vi "Server.vi"() -> ()   [LabVIEW 2021]
panel:
  out "MasterBedRoomD":u8(slide) scale=0.0..100.0
  out "Balcony2D":u8(slide) scale=0.0..100.0
  out "KitchenToiletD":u8(slide) scale=0.0..100.0
  out "Balcony1D2":u8(slide) scale=0.0..100.0
  out "LivingRoomD":u8(slide) scale=0.0..100.0
  out "LRToiletD":u8(slide) scale=0.0..100.0
  out "KitchenD":u8(slide) scale=0.0..100.0
  out "Balcony1D1":u8(slide) scale=0.0..100.0
  out "MBToiletD":u8(slide) scale=0.0..100.0
  out "Bedroom1D":u8(slide) scale=0.0..100.0
  out "Bedroom2D":u8(slide) scale=0.0..100.0
  out "MasterBedroomL2":bool
  out "MasterBedroomL1":bool
  out "LivingRoomL2":bool
  out "Bedroom1L":bool
  out "Bedroom2L":bool
  out "LRToiletL":bool
  out "LivingRoomL1":bool
  out "KitchenToiletL":bool
  out "KitchenL":bool
  out "BalconyL3":bool
  out "BalconyL2":bool
  out "BalconyL1":bool
  out "LivingRoomC":u8(slide) scale=0.0..10.0
  out "MasterBedroomC":u8(slide) scale=0.0..10.0
  in  "WindowsMediaPlayer":refnum<k7>(container)
  out "Electric Usage":dbl(knob) scale=0.0..100.0
  # "Balcony 2"
  # "TV"
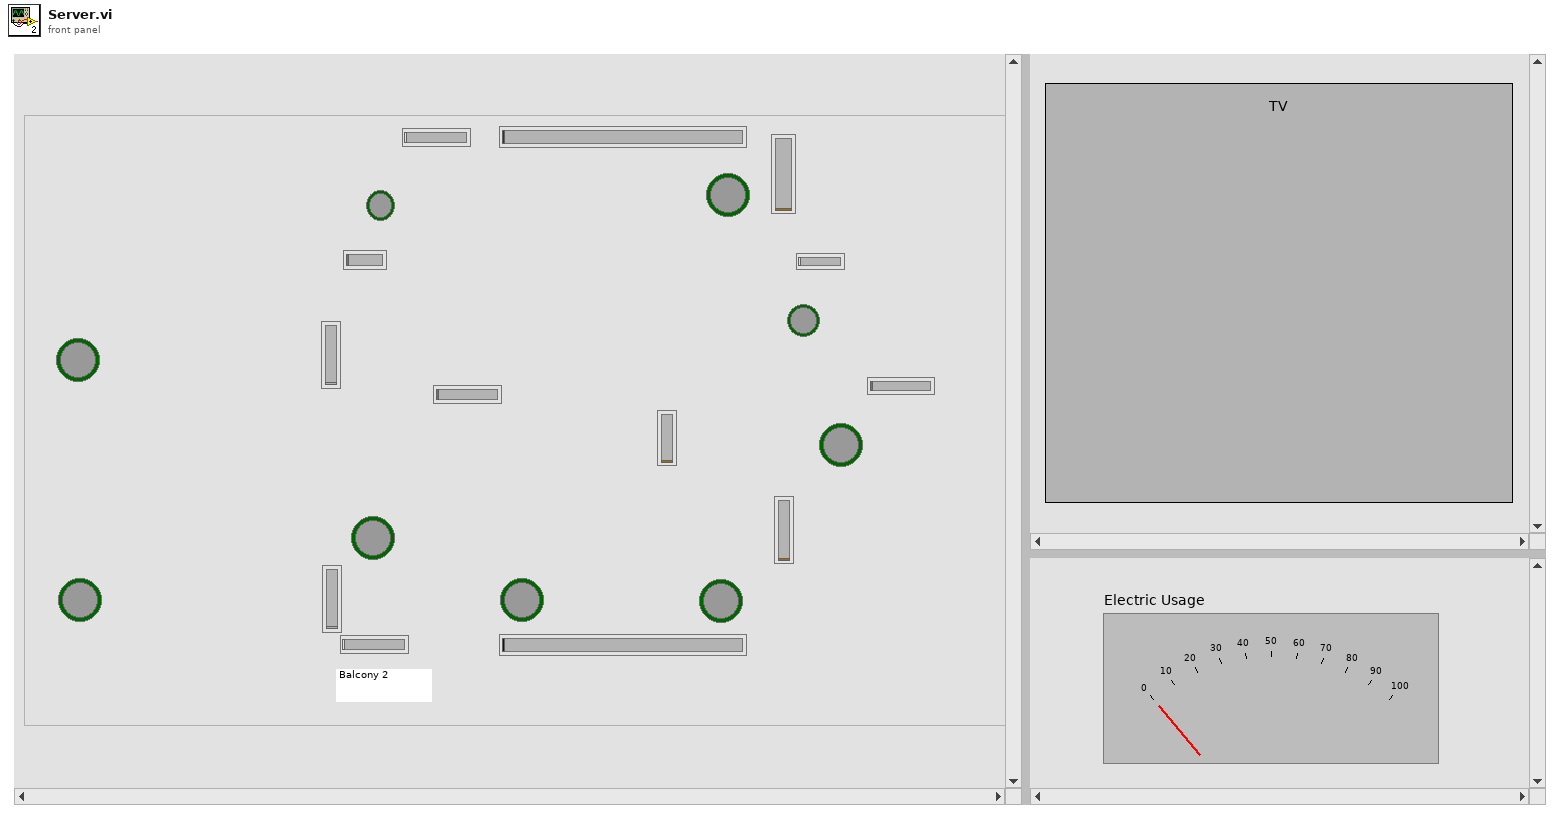
[diagram p1: front panel]
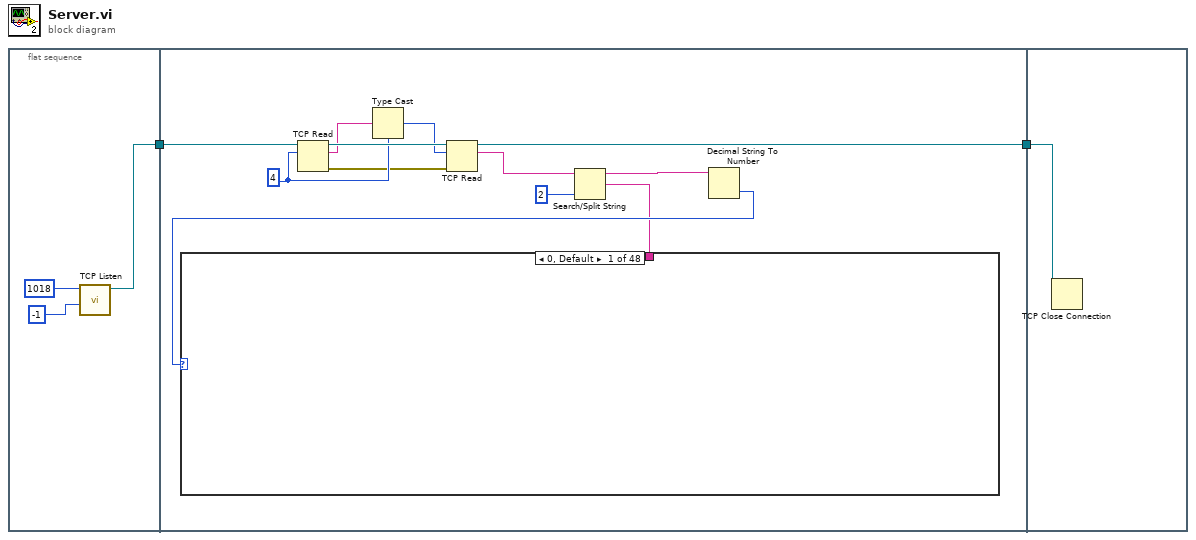
[diagram p0: block diagram]
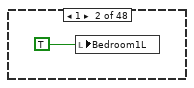
[diagram p2: hidden frame]
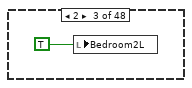
[diagram p3: hidden frame]
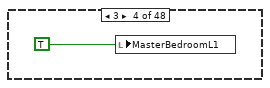
[diagram p4: hidden frame]
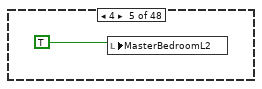
[diagram p5: hidden frame]
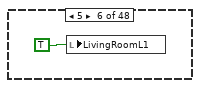
[diagram p6: hidden frame]
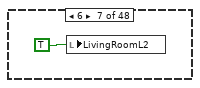
[diagram p7: hidden frame]
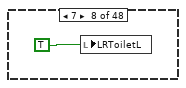
[diagram p8: hidden frame]
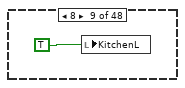
[diagram p9: hidden frame]
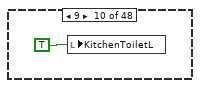
[diagram p10: hidden frame]
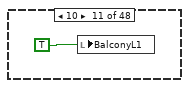
[diagram p11: hidden frame]
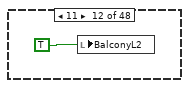
[diagram p12: hidden frame]
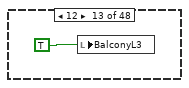
[diagram p13: hidden frame]
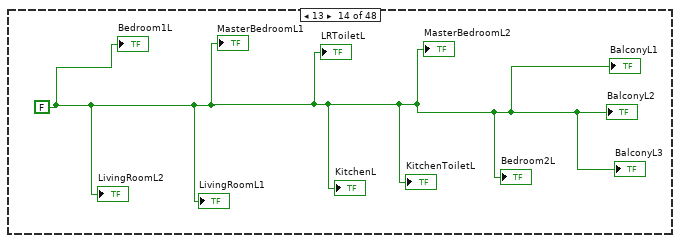
[diagram p14: hidden frame]
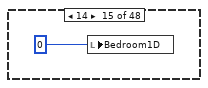
[diagram p15: hidden frame]
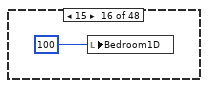
[diagram p16: hidden frame]
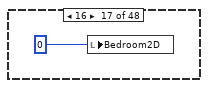
[diagram p17: hidden frame]
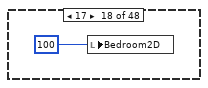
[diagram p18: hidden frame]
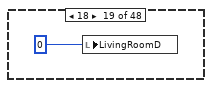
[diagram p19: hidden frame]
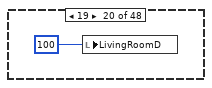
[diagram p20: hidden frame]
diagram:
  n1 = flat-sequence {
    tunnel: [w4] -> w2
    tunnel: w2 -> [w13]
    tunnel: [w12] -> w1
    tunnel: w1 -> [w95]
    frame #0 {
      n2 = call <vilib>:"TCP Listen.vi"("timeout ms (wait forever: -1)"=-1, "port"=1018) -> ("connection ID"=w4:refnum<k5>)  [unwired: 5 in, 4 out]
    }
    frame #1 {
      w11 = 4
      n3 = TCP Read(connection ID=w13, bytes to read=w11) -> (connection ID out=w17:refnum<k5>, data out=w15:string, error out=w6:errorcluster)  [unwired: 3 in]
      n4 = Type Cast(type=w11, x=w15) -> (*(type *) &x=w16:i32)
      n5 = TCP Read(connection ID=w17, bytes to read=w16, error in (no error)=w6) -> (connection ID out=w12:refnum<k5>, data out=w8:string)  [unwired: 2 in, 1 out]
      n6 = Search/Split String(string=w8, offset (0)=2) -> (substring before match=w7:string, match + rest of string=w9:string)  [unwired: 1 in, 1 out]
      n7 = Decimal String To Number(string=w7) -> (number=w10:i32)  [unwired: 2 in, 1 out]
      n8 = case shown="0, Default" w10 {
        tunnel: w9 -> [_ _ _ _ _ _ _ _ _ _ _ _ _ _ _ _ _ _ _ _ _ _ _ _ _ _ _ _ _ _ _ _ _ _ _ _ _ w55 w57 _ _ _ _ _ _ w82 w93 _]
        frame 0, Default {
        }
        frame 1 {
          n9 = local write "Bedroom1L"(TRUE) -> ()
        }
        frame 2 {
          n10 = local write "Bedroom2L"(TRUE) -> ()
        }
        frame 3 {
          n11 = local write "MasterBedroomL1"(TRUE) -> ()
        }
        frame 4 {
          n12 = local write "MasterBedroomL2"(TRUE) -> ()
        }
        frame 5 {
          n13 = local write "LivingRoomL1"(TRUE) -> ()
        }
        frame 6 {
          n14 = local write "LivingRoomL2"(TRUE) -> ()
        }
        frame 7 {
          n15 = local write "LRToiletL"(TRUE) -> ()
        }
        frame 8 {
          n16 = local write "KitchenL"(TRUE) -> ()
        }
        frame 9 {
          n17 = local write "KitchenToiletL"(TRUE) -> ()
        }
        frame 10 {
          n18 = local write "BalconyL1"(TRUE) -> ()
        }
        frame 11 {
          n19 = local write "BalconyL2"(TRUE) -> ()
        }
        frame 12 {
          n20 = local write "BalconyL3"(TRUE) -> ()
        }
        frame 13 {
          w30 = FALSE
          "BalconyL1" <- w30
          "KitchenToiletL" <- w30
          "LivingRoomL1" <- w30
          "LRToiletL" <- w30
          "Bedroom1L" <- w30
          "LivingRoomL2" <- w30
          "MasterBedroomL1" <- w30
          "MasterBedroomL2" <- w30
          "BalconyL3" <- w30
          "KitchenL" <- w30
          "BalconyL2" <- w30
          "Bedroom2L" <- w30
        }
        frame 14 {
          n21 = local write "Bedroom1D"(0) -> ()
        }
        frame 15 {
          n22 = local write "Bedroom1D"(100) -> ()
        }
        frame 16 {
          n23 = local write "Bedroom2D"(0) -> ()
        }
        frame 17 {
          n24 = local write "Bedroom2D"(100) -> ()
        }
        frame 18 {
          n25 = local write "LivingRoomD"(0) -> ()
        }
        frame 19 {
          n26 = local write "LivingRoomD"(100) -> ()
        }
        frame 20 {
          n27 = local write "LRToiletD"(0) -> ()
        }
        frame 21 {
          n28 = local write "LRToiletD"(100) -> ()
        }
        frame 22 {
          n29 = local write "MasterBedRoomD"(0) -> ()
        }
        frame 23 {
          n30 = local write "MasterBedRoomD"(100) -> ()
        }
        frame 24 {
          n31 = local write "MBToiletD"(0) -> ()
        }
        frame 25 {
          n32 = local write "MBToiletD"(100) -> ()
        }
        frame 26 {
          n33 = local write "KitchenD"(0) -> ()
        }
        frame 27 {
          n34 = local write "KitchenD"(100) -> ()
        }
        frame 28 {
          n35 = local write "KitchenToiletD"(0) -> ()
        }
        frame 29 {
          n36 = local write "KitchenToiletD"(100) -> ()
        }
        frame 30 {
          n37 = local write "Balcony1D1"(0) -> ()
        }
        frame 31 {
          n38 = local write "Balcony1D1"(100) -> ()
        }
        frame 32 {
          n39 = local write "Balcony1D2"(0) -> ()
        }
        frame 33 {
          n40 = local write "Balcony1D2"(100) -> ()
        }
        frame 34 {
          n41 = local write "Balcony2D"(0) -> ()
        }
        frame 35 {
          n42 = local write "Balcony2D"(100) -> ()
        }
        frame 36 {
          w53 = 100
          "Balcony2D" <- w53
          "Bedroom1D" <- w53
          "Bedroom2D" <- w53
          "MasterBedRoomD" <- w53
          "MBToiletD" <- w53
          "Balcony1D1" <- w53
          "Balcony1D2" <- w53
          "LRToiletD" <- w53
          "LivingRoomD" <- w53
          "KitchenD" <- w53
          "KitchenToiletD" <- w53
        }
        frame 37 {
          n43 = Decimal String To Number(string=w55) -> (number=→"LivingRoomC":i32)  [unwired: 2 in, 1 out]
        }
        frame 38 {
          n44 = Decimal String To Number(string=w57) -> (number=→"MasterBedroomC":i32)  [unwired: 2 in, 1 out]
        }
        frame 39 {
          n45 = Automation Open(Automation Refnum="WindowsMediaPlayer") -> (Automation Refnum=w60:refnum<k7>)  [unwired: 3 in, 1 out]
          n46 = property class="IWMPPlayer4"(reference=w60) -> ("controls"=w59:refnum<k7>)  [unwired: 1 in, 2 out]
          n47 = invoke class="IWMPControls" method="stop"(reference=w59) -> (reference out=w58:refnum<k7>)  [unwired: 2 in, 2 out]
          n48 = Close Reference(reference=w58) -> ()  [unwired: 1 in, 1 out]
        }
        frame 40 {
          # "Pause"
          n49 = local read "WindowsMediaPlayer"() -> (w62:refnum<k7>)
          n50 = Automation Open(Automation Refnum=w62) -> (Automation Refnum=w63:refnum<k7>)  [unwired: 3 in, 1 out]
          n51 = property class="IWMPPlayer4"(reference=w63) -> ("controls"=w64:refnum<k7>)  [unwired: 1 in, 2 out]
          n52 = invoke class="IWMPControls" method="pause"(reference=w64) -> (reference out=w65:refnum<k7>)  [unwired: 2 in, 2 out]
          n53 = Close Reference(reference=w65) -> ()  [unwired: 1 in, 1 out]
        }
        frame 41 {
          # "Channel1"
          n54 = local read "WindowsMediaPlayer"() -> (w67:refnum<k7>)
          n55 = Automation Open(Automation Refnum=w67) -> (Automation Refnum=w68:refnum<k7>)  [unwired: 3 in, 1 out]
          n56 = property class="IWMPPlayer4"(reference=w68, "URL"="D:\\APU\\Academics\\Degree\\Year 2 - Sem 1\\spcc\\Assignment\\Submission\\YamChenXi_TP061635\\Materials\\Advert.mp4") -> (reference out=w69:refnum<k7>)  [unwired: 1 in, 1 out]
          n57 = Close Reference(reference=w69) -> ()  [unwired: 1 in, 1 out]
        }
        frame 42 {
          # "Channel2"
          n58 = local read "WindowsMediaPlayer"() -> (w73:refnum<k7>)
          n59 = Automation Open(Automation Refnum=w73) -> (Automation Refnum=w72:refnum<k7>)  [unwired: 3 in, 1 out]
          n60 = property class="IWMPPlayer4"(reference=w72, "URL"="D:\\APU\\Academics\\Degree\\Year 2 - Sem 1\\spcc\\Assignment\\Submission\\YamChenXi_TP061635\\Materials\\Wildlife.mp4") -> (reference out=w71:refnum<k7>)  [unwired: 1 in, 1 out]
          n61 = Close Reference(reference=w71) -> ()  [unwired: 1 in, 1 out]
        }
        frame 43 {
          # "Channel3"
          n62 = local read "WindowsMediaPlayer"() -> (w77:refnum<k7>)
          n63 = Automation Open(Automation Refnum=w77) -> (Automation Refnum=w76:refnum<k7>)  [unwired: 3 in, 1 out]
          n64 = property class="IWMPPlayer4"(reference=w76, "URL"="D:\\APU\\Academics\\Degree\\Year 2 - Sem 1\\spcc\\Assignment\\Submission\\YamChenXi_TP061635\\Materials\\CuriousCat.mp4") -> (reference out=w75:refnum<k7>)  [unwired: 1 in, 1 out]
          n65 = Close Reference(reference=w75) -> ()  [unwired: 1 in, 1 out]
        }
        frame 44 {
          # "Play"
          n66 = local read "WindowsMediaPlayer"() -> (w81:refnum<k7>)
          n67 = Automation Open(Automation Refnum=w81) -> (Automation Refnum=w80:refnum<k7>)  [unwired: 3 in, 1 out]
          n68 = property class="IWMPPlayer4"(reference=w80) -> ("controls"=w79:refnum<k7>)  [unwired: 1 in, 2 out]
          n69 = invoke class="IWMPControls" method="play"(reference=w79) -> (reference out=w78:refnum<k7>)  [unwired: 2 in, 2 out]
          n70 = Close Reference(reference=w78) -> ()  [unwired: 1 in, 1 out]
        }
        frame 45 {
          # "Volume"
          n71 = local read "WindowsMediaPlayer"() -> (w87:refnum<k7>)
          n72 = Automation Open(Automation Refnum=w87) -> (Automation Refnum=w83:refnum<k7>)  [unwired: 3 in, 1 out]
          n73 = property class="IWMPPlayer4"(reference=w83) -> ("settings"=w84:refnum<k7>)  [unwired: 1 in, 2 out]
          n74 = Decimal String To Number(string=w82) -> (number=w85:i32)  [unwired: 2 in, 1 out]
          n75 = property class="IWMPSettings"(reference=w84, "volume"=w85) -> (reference out=w86:refnum<k7>)  [unwired: 1 in, 1 out]
          n76 = Close Reference(reference=w86) -> ()  [unwired: 1 in, 1 out]
        }
        frame 46 {
          n77 = Decimal String To Number(string=w93) -> (number=w92:i32)  [unwired: 2 in, 1 out]
          n78 = Multiply(x=w92, y=100) -> (x*y=w90:i32)
          n79 = Divide(x=w90, y=12) -> (x/y=→"Electric Usage":dbl)
        }
        frame 47 {
          w94 = 0
          n80 = local write "Balcony1D2"(w94) -> ()
          n81 = local write "Balcony1D1"(w94) -> ()
          n82 = local write "Bedroom1D"(w94) -> ()
          n83 = local write "Balcony2D"(w94) -> ()
          n84 = local write "Bedroom2D"(w94) -> ()
          n85 = local write "KitchenD"(w94) -> ()
          n86 = local write "KitchenToiletD"(w94) -> ()
          n87 = local write "LRToiletD"(w94) -> ()
          n88 = local write "LivingRoomD"(w94) -> ()
          n89 = local write "MBToiletD"(w94) -> ()
          n90 = local write "MasterBedRoomD"(w94) -> ()
        }
      }
    }
    frame #2 {
      n91 = TCP Close Connection(connection ID=w95) -> ()  [unwired: 2 in, 2 out]
    }
  }
